vi "Page Engine.vi"(7 "Action":T5, 8 "error in (no error)":errorcluster, 11 "Data in":variant) -> (0 "error out":errorcluster, 3 "Data out":variant)   [LabVIEW 2018, in "Page.lvlib"]
uses:
  Page.lvlib
  Page Refnums.ctl
  Page Action.ctl
  Page Mouse.ctl
  <vilib>/Utility/miscctls.llb/LVPoint32TypeDef.ctl
  <vilib>/Utility/miscctls.llb/LVPointTypeDef.ctl
  Page Add.ctl
  Theme/Theme Colors.vi
  Theme/Theme.lvlib
  <vilib>/picture/picture.llb/imagedata.ctl
panel:
  in  "StateData":T4={"Refnums"={"VI Refnum"=refnum, "Sub Panel"=refnum, "Picture"=refnum}, "Page"={"Height"=32, "ActiveIdx"=0, "HoverIdx"=0, "Mouse"={"Horizontal"=0, "Vertical"=0, "Button"=0, "Shift"=FALSE, "Ctrl"=FALSE, "Alt"=FALSE, "Double Click"=FALSE}}, "Pages"={"VI Refnums"=[], "Captions"=[], "Titles"=[], "Images"=[], "Running"=[]}, "Ready"=FALSE}
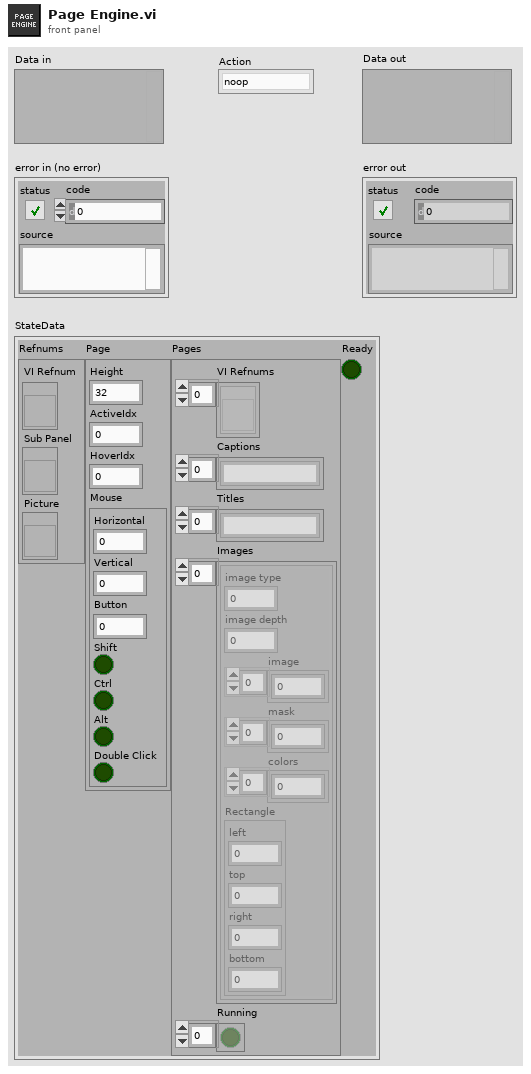
[diagram p1: front panel]
types:
  T1 = typedef "Page.lvlib/Page Refnums.ctl" = cluster{"VI Refnum":refnum<vi>, "Sub Panel":refnum<vi>, "Picture":refnum<vi>}
  T2 = typedef "Page.lvlib/Page Mouse.ctl" = cluster{"Horizontal":i32, "Vertical":i32, "Button":u16, "Shift":bool, "Ctrl":bool, "Alt":bool, "Double Click":bool}
  T3 = typedef "imagedata.ctl" = cluster{"image type":i32, "image depth":i32, "image":u8[], "mask":u8[], "colors":u32[], "Rectangle":cluster{"left":i16, "top":i16, "right":i16, "bottom":i16}}
  T4 = cluster{"Refnums":T1, "Page":cluster{"Height":i32, "ActiveIdx":i32, "HoverIdx":i32, "Mouse":T2}, "Pages":cluster{"VI Refnums":refnum<vi>[], "Captions":string[], "Titles":string[], "Images":T3[], "Running":bool[]}, "Ready":bool}
  T5 = typedef "Page.lvlib/Page Action.ctl" = enum8{"noop", "new", "init", "close", "page_change", "page_hover", "render", "page_caption", "page_insert", "page_add", "start", "resize", "theme_change", "hide"}
  T6 = typedef "LVPointTypeDef.ctl" = cluster{"Horizontal":i16, "Vertical":i16}
  T7 = typedef "LVPoint32TypeDef.ctl" = cluster{"Horizontal":i32, "Vertical":i32}
  T8 = cluster{"left":i16, "top":i16, "right":i16, "bottom":i16}
  T9 = typedef "Page.lvlib/Page Add.ctl" = cluster{"VI Path":path, "Caption":string}
  T10 = enum32{"Invalid", "Standard", "Closed", "Hidden", "Minimized", "Maximized"}
  T11 = typedef "LVRectTypeDef.ctl" = cluster{"Left":i16, "Top":i16, "Right":i16, "Bottom":i16}
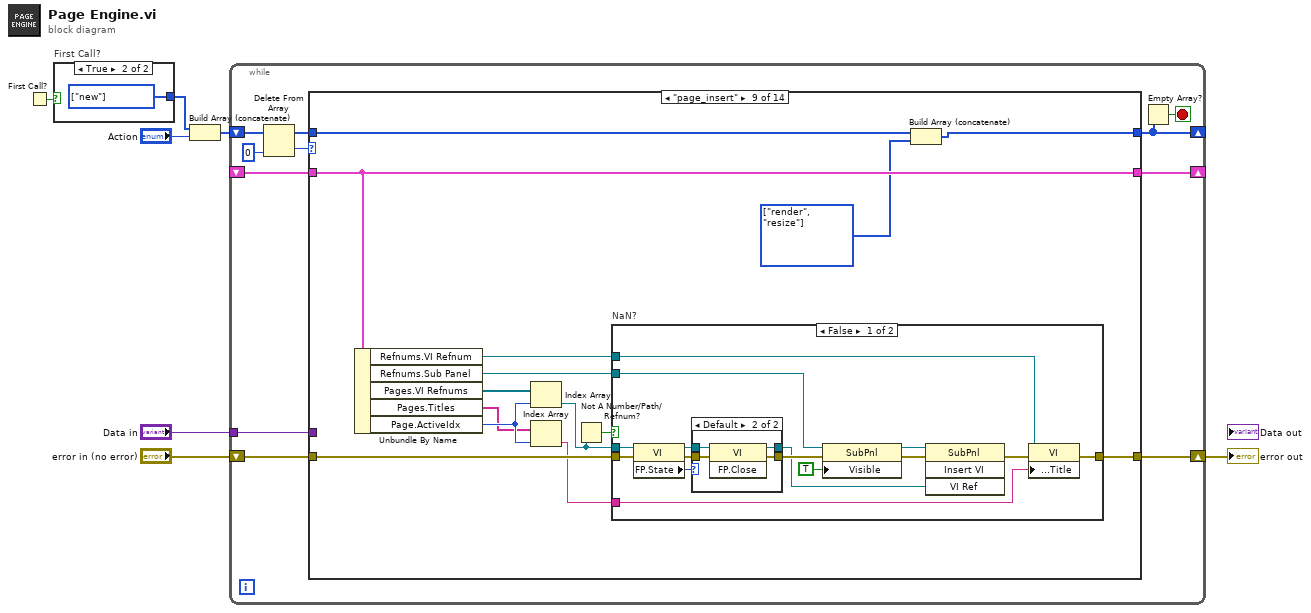
[diagram p0: block diagram]
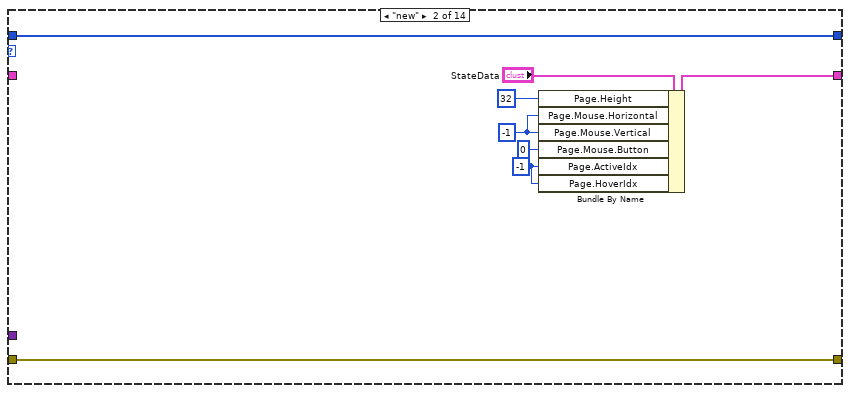
[diagram p4: hidden frame]
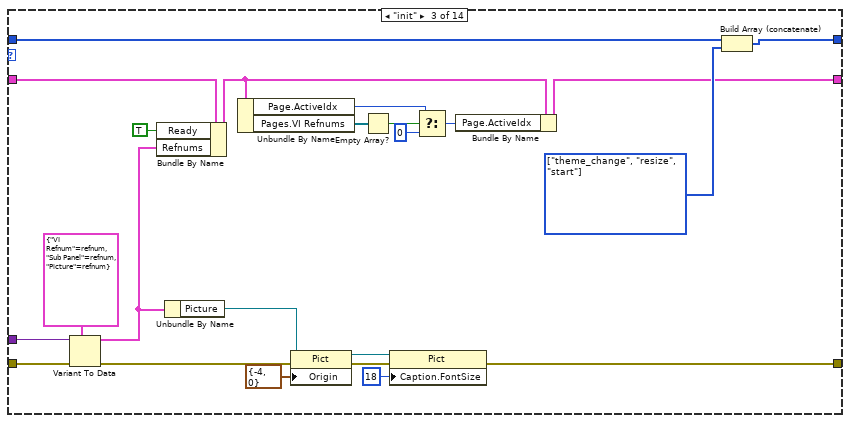
[diagram p5: hidden frame]
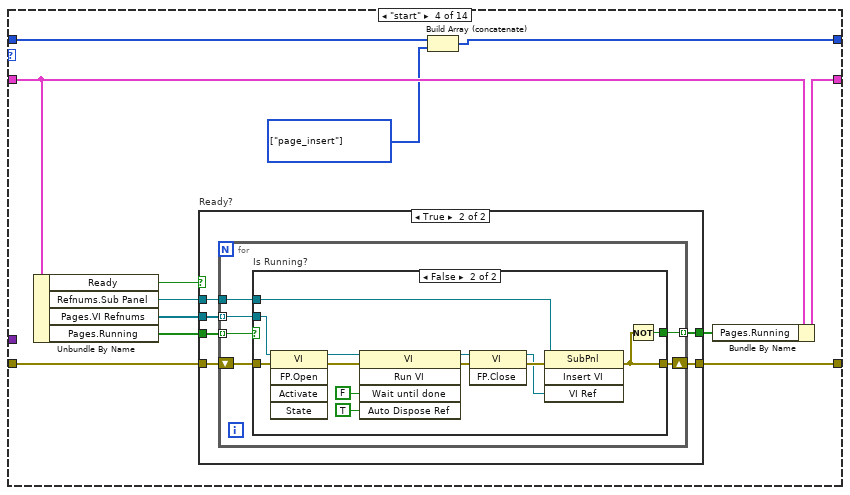
[diagram p6: hidden frame]
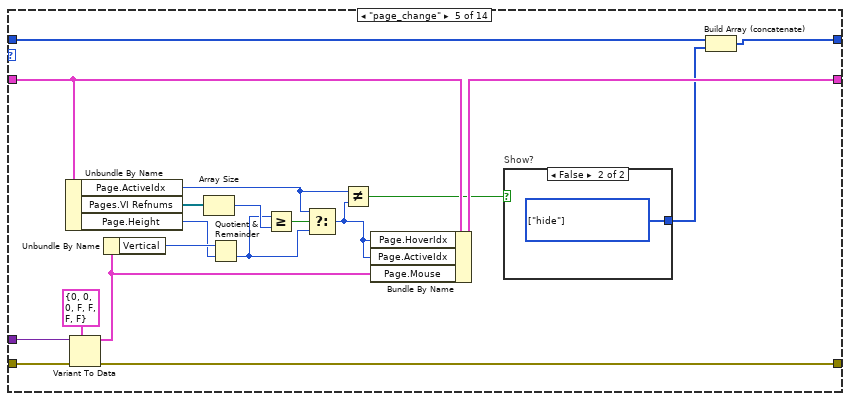
[diagram p9: hidden frame]
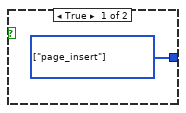
[diagram p10: hidden frame]
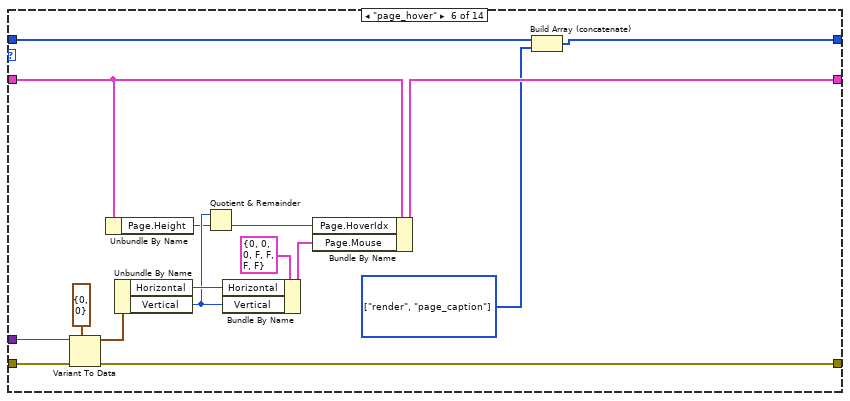
[diagram p11: hidden frame]
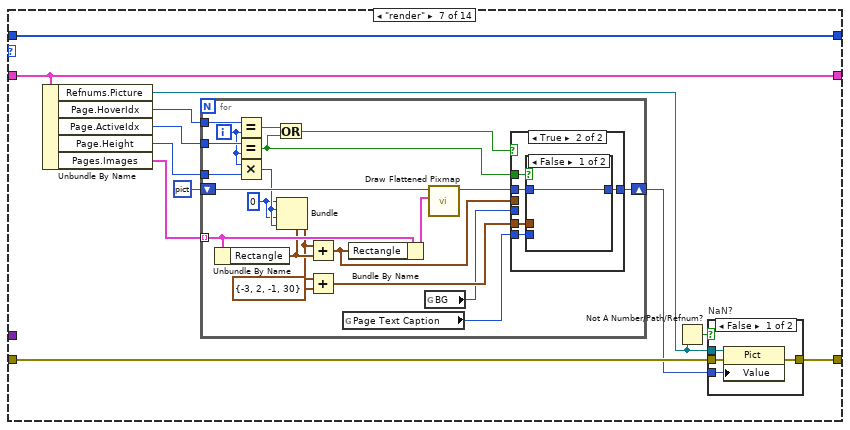
[diagram p12: hidden frame]
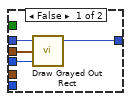
[diagram p14: hidden frame]
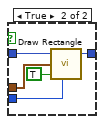
[diagram p15: hidden frame]
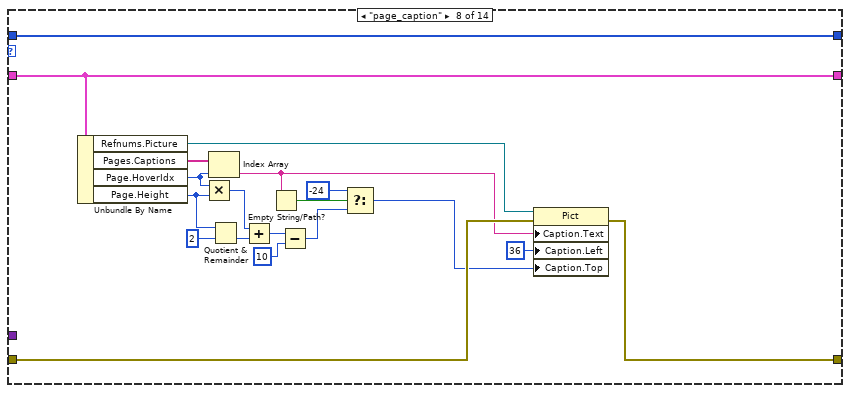
[diagram p16: hidden frame]
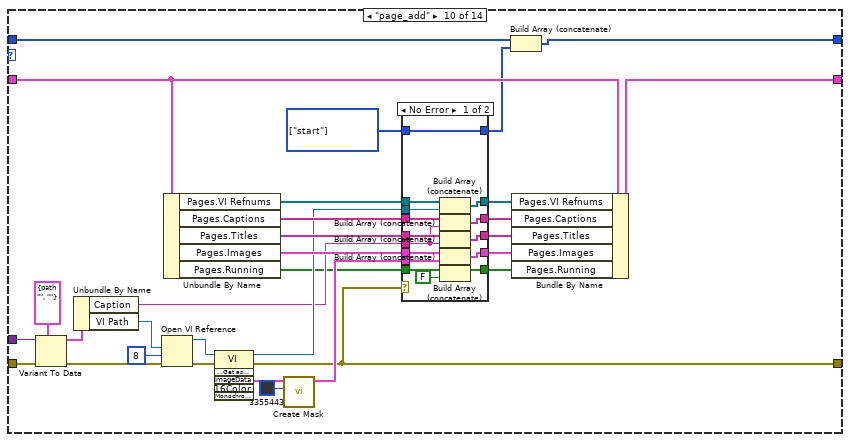
[diagram p19: hidden frame]
diagram:
  n1 = First Call?() -> (First Call?: T/F=w1:bool)
  n2 = case "First Call?" shown="True" w1 {
    tunnel: [_ w8] -> w2
    frame False {
    }
    frame True {
      w8 = T5[] [enum."new"] items=["noop", "new", "init", "close", "page_change", "page_hover", "render", "page_caption", "page_insert", "page_add", "start", "resize", "theme_change", "hide"] ("element")
    }
  }
  n3 = Build Array (concatenate)(w2, "Action") -> (w3:T5[])
  n4 = while {
    tunnel: "Data in" -> [w17]
    shift-right: [w18] -> w6
    shift-left: "error in (no error)" -> [w19]
    shift-right: [w12] -> _
    shift-left: w3 -> [w16]
    shift-right: [w10] -> _
    shift-left: _ -> [w9]
    stop <- w11 stop-if-true
    n5 = Delete From Array(array=w16, index=0) -> (deleted portion=w13:T5, array with subset deleted=w15:T5[])  [unwired: 1 in]
    n6 = case shown="\"page_insert\"" w13 {
      tunnel: w19 -> [w21 w30 w53 w62 w113 w131 w140 w196 w217 w270 w291 w317 w322 w362]
      tunnel: [w21 w30 w40 w63 w112 w130 w141 w197 w213 w248 w291 w306 w326 w355] -> w18
      tunnel: w17 -> [_ _ w51 _ w111 w129 _ _ _ w267 _ _ _ _]
      tunnel: w15 -> [w22 w29 w49 w65 w110 w128 w143 w203 w216 w269 w293 w316 w328 w361]
      tunnel: [w22 w29 w47 w58 w108 w126 w143 w203 w211 w247 w293 w316 w319 w358] -> w12
      tunnel: [w20 w27 w32 w55 w109 w127 w142 w202 w215 w262 w292 w315 w327 w360] -> w10
      tunnel: w9 -> [w20 _ w48 w64 w104 w124 w142 w202 w215 w263 w292 w315 w327 w356]
      frame "noop" {
      }
      frame "new" {
        w23 = -1 ("Page.ActiveIdx")
        w25 = -1 ("Page Mouse.Vertical")
        n7 = Bundle By Name(cluster="StateData", "Page.Height"=32 ("PageHeight"), "Page.Mouse.Horizontal"=w25, "Page.Mouse.Vertical"=w25, "Page.Mouse.Button"=u16 0, "Page.ActiveIdx"=w23, "Page.HoverIdx"=w23) -> (w27:T4)
      }
      frame "init" {
        w46 = T5[] [enum."theme_change", enum."resize", enum."start"] items=["noop", "new", "init", "close", "page_change", "page_hover", "render", "page_caption", "page_insert", "page_add", "start", "resize", "theme_change", "hide"] ("array")
        n8 = Variant To Data(error in=w53, type=T1 {"VI Refnum"=refnum, "Sub Panel"=refnum, "Picture"=refnum} ("Refnums"), Variant=w51) -> (data=w45:T1, error out=w52:errorcluster)
        n9 = Bundle By Name(cluster=w48, "Ready"=TRUE, "Refnums"=w45) -> (w37:T4)
        n10 = Unbundle By Name(w45) -> ("Picture"=w43:refnum<vi>)
        n11 = Unbundle By Name(w37) -> ("Page.ActiveIdx"=w34:i32, "Pages.VI Refnums"=w36:refnum<vi>[])
        n12 = property class="Pict"(reference=w43, error in=w52, "Origin"=T6 {"Horizontal"=-4, "Vertical"=0}) -> (reference out=w39:refnum<vi>, error out=w44:errorcluster)
        n13 = Empty Array?(array=w36) -> (empty?=w35:bool)
        n14 = property class="Pict"(reference=w39, error in=w44, "Caption.FontSize"=u32 18 ("Caption.Font:Size")) -> (error out=w40:errorcluster)  [unwired: 1 out]
        n15 = Select(t=w34, s=w35, f=0) -> (s? t:f=w31:i32)
        n16 = Bundle By Name(cluster=w37, "Page.ActiveIdx"=w31) -> (w32:T4)
        n17 = Build Array (concatenate)(w49, w46) -> (w47:T5[])
      }
      frame "start" {
        w57 = T5[] [enum."page_insert"] items=["noop", "new", "init", "close", "page_change", "page_hover", "render", "page_caption", "page_insert", "page_add", "start", "resize", "theme_change", "hide"] ("array")
        n18 = Unbundle By Name(w64) -> ("Ready"=w59:bool, "Refnums.Sub Panel"=w60:refnum<vi>, "Pages.VI Refnums"=w61:refnum<vi>[], "Pages.Running"=w56:bool[])
        n19 = case "Ready?" shown="True" w59 {
          tunnel: [w67 w73] -> w63
          tunnel: w62 -> [w67 w72]
          tunnel: w61 -> [_ w71]
          tunnel: w60 -> [_ w70]
          tunnel: w56 -> [w66 w69]
          tunnel: [w66 w68] -> w54
          frame False {
          }
          frame True {
            n20 = for {
              tunnel: w71 -> [w77] mode=indexing
              shift-right: [w79] -> w73
              shift-left: w72 -> [w76]
              tunnel: w70 -> [w78]
              tunnel: w69 -> [w75] mode=indexing
              tunnel: [w74] -> w68 mode=indexing
              n21 = case "Is Running?" shown="False" w75 {
                selector: w75 -> [w80 _]
                tunnel: w76 -> [w81 w87]
                tunnel: w77 -> [_ w86]
                tunnel: [w81 w83] -> w79
                tunnel: w78 -> [_ w85]
                tunnel: [w80 w82] -> w74
                frame True {
                }
                frame False {
                  n22 = invoke class="VI" method="FP.Open"(reference=w86, error in=w87) -> (reference out=w90:refnum<vi>, error out=w91:errorcluster)  [unwired: 3 in, 3 out]
                  n23 = invoke class="VI" method="Run VI"(reference=w90, error in=w91, "Wait until done"=FALSE ("Wait Until Done"), "Auto Dispose Ref"=TRUE ("Auto Dispose Reference")) -> (reference out=w89:refnum<vi>, error out=w94:errorcluster)  [unwired: 1 in, 3 out]
                  n24 = invoke class="VI" method="FP.Close"(reference=w89, error in=w94) -> (reference out=w84:refnum<vi>, error out=w88:errorcluster)  [unwired: 1 in, 1 out]
                  n25 = invoke class="SubPnl" method="Insert VI"(reference=w85, error in=w88, "VI Ref"=w84) -> (error out=w83:errorcluster)  [unwired: 1 in, 3 out]
                  n26 = Not(x=w83) -> (.not. x?=w82:bool)
                }
              }
            }
          }
        }
        n27 = Build Array (concatenate)(w65, w57) -> (w58:T5[])
        n28 = Bundle By Name(cluster=w64, "Pages.Running"=w54) -> (w55:T4)
      }
      frame "page_change" {
        n29 = Unbundle By Name(w104) -> ("Page.ActiveIdx"=w96:i32, "Pages.VI Refnums"=w101:refnum<vi>[], "Page.Height"=w102:i32)
        n30 = Variant To Data(error in=w113, type=T2 {"Horizontal"=0, "Vertical"=0, "Button"=0, "Shift"=FALSE, "Ctrl"=FALSE, "Alt"=FALSE, "Double Click"=FALSE} ("Page Mouse"), Variant=w111) -> (data=w105:T2, error out=w112:errorcluster)
        n31 = Unbundle By Name(w105) -> ("Vertical"=w103:i32)
        n32 = Array Size(array=w101) -> (size(s)=w100:i32)
        n33 = Quotient & Remainder(x=w103, y=w102) -> (floor(x/y)=w98:i32)  [unwired: 1 out]
        n34 = Greater Or Equal?(x=w98, y=w100) -> (x >= y?=w99:bool)
        n35 = Select(t=w96, s=w99, f=w98) -> (s? t:f=w97:i32)
        n36 = Not Equal?(x=w96, y=w97) -> (x != y?=w95:bool)
        n37 = Bundle By Name(cluster=w104, "Page.HoverIdx"=w97, "Page.ActiveIdx"=w97, "Page.Mouse"=w105) -> (w109:T4)
        n38 = case "Show?" shown="False" w95 {
          tunnel: [w114 w115] -> w107
          frame True {
            w114 = T5[] [enum."page_insert"] items=["noop", "new", "init", "close", "page_change", "page_hover", "render", "page_caption", "page_insert", "page_add", "start", "resize", "theme_change", "hide"] ("array")
          }
          frame False {
            w115 = T5[] [enum."hide"] items=["noop", "new", "init", "close", "page_change", "page_hover", "render", "page_caption", "page_insert", "page_add", "start", "resize", "theme_change", "hide"] ("array")
          }
        }
        n39 = Build Array (concatenate)(w110, w107) -> (w108:T5[])
      }
      frame "page_hover" {
        w125 = T5[] [enum."render", enum."page_caption"] items=["noop", "new", "init", "close", "page_change", "page_hover", "render", "page_caption", "page_insert", "page_add", "start", "resize", "theme_change", "hide"] ("array")
        n40 = Variant To Data(error in=w131, type=T7 {"Horizontal"=0, "Vertical"=0} ("Coords"), Variant=w129) -> (data=w120:T7, error out=w130:errorcluster)
        n41 = Unbundle By Name(w124) -> ("Page.Height"=w117:i32)
        n42 = Unbundle By Name(w120) -> ("Horizontal"=w119:i32, "Vertical"=w118:i32)
        n43 = Quotient & Remainder(x=w118, y=w117) -> (floor(x/y)=w116:i32)  [unwired: 1 out]
        n44 = Bundle By Name(cluster=T2 {"Horizontal"=0, "Vertical"=0, "Button"=0, "Shift"=FALSE, "Ctrl"=FALSE, "Alt"=FALSE, "Double Click"=FALSE} ("Page.Mouse"), "Horizontal"=w119, "Vertical"=w118) -> (w122:T2)
        n45 = Bundle By Name(cluster=w124, "Page.HoverIdx"=w116, "Page.Mouse"=w122) -> (w127:T4)
        n46 = Build Array (concatenate)(w128, w125) -> (w126:T5[])
      }
      frame "render" {
        n47 = Unbundle By Name(w142) -> ("Refnums.Picture"=w133:refnum<vi>, "Page.HoverIdx"=w137:i32, "Page.ActiveIdx"=w138:i32, "Page.Height"=w135:i32, "Pages.Images"=w139:T3[])
        n48 = for {
          tunnel: w139 -> [w168] mode=indexing
          tunnel: w138 -> [w169]
          tunnel: w137 -> [w166]
          shift-right: [w164] -> w134
          shift-left: picture data[5B] ("new picture") -> [w163]
          tunnel: w135 -> [w160]
          i -> [w161]
          w157 = i16 0 ("left")
          n49 = Unbundle By Name(w168) -> ("Rectangle"=w162:T8)
          n50 = Equal?(x=w166, y=w161) -> (x = y?=w158:bool)
          n51 = Equal?(x=w169, y=w161) -> (x = y?=w151:bool)
          n52 = Multiply(x=w161, y=w160) -> (x*y=w159:i32)
          n53 = Or(x=w158, y=w151) -> (x .or. y?=w152:bool)
          n54 = Bundle(cluster=w162, "left"=w157, "top"=w159, "right"=w157, "bottom"=w159) -> (w155:T8)
          n55 = Add(x=w155, y=w162) -> (x+y=w156:T8)
          n56 = Add(x=w155, y=T8 {"left"=-3, "top"=2, "right"=-1, "bottom"=30}) -> (x+y=w153:T8)
          n57 = global read "Theme Colors.vi" "Page Text Caption"() -> (w149:u32)
          n58 = Bundle By Name(cluster=w168, "Rectangle"=w156) -> (w167:T3)
          n59 = global read "Theme Colors.vi" "BG"() -> (w150:u32)
          n60 = call <vilib>:"Draw Flattened Pixmap.vi"("image data"=w167, "picture"=w163) -> ("new picture"=w165:picture)  [unwired: 7 in]
          n61 = case shown="True" w152 {
            tunnel: w150 -> [w173 _]
            tunnel: w165 -> [w172 w178]
            tunnel: w156 -> [w171 _]
            tunnel: [w170 w177] -> w164
            tunnel: w153 -> [_ w176]
            tunnel: w149 -> [_ w175]
            tunnel: w151 -> [_ w174]
            frame False {
              n62 = call <vilib>:"Draw Grayed Out Rect.vi"("color(black)"=w173, "rect"=w171, "picture"=w172) -> ("new picture"=w170:picture)  [unwired: 2 in]
            }
            frame True {
              n63 = case shown="False" w174 {
                tunnel: w178 -> [w179 w184]
                tunnel: [w179 w183] -> w177
                tunnel: w176 -> [_ w182]
                tunnel: w175 -> [_ w180]
                frame False {
                }
                frame True {
                  n64 = call <vilib>:"Draw Rectangle.vi"("picture"=w184, "rect"=w182, "fill?(F)"=TRUE, "color(black)"=w180) -> ("new picture"=w183:picture)  [unwired: 5 in]
                }
              }
            }
          }
        }
        n65 = Not A Number/Path/Refnum?(number/path/refnum=w133) -> (NaN/Path/Refnum?=w132:bool)
        n66 = case "NaN?" shown="False" w132 {
          tunnel: w133 -> [w147 _]
          tunnel: [w146 w148] -> w141
          tunnel: w140 -> [w145 w148]
          tunnel: w134 -> [w144 _]
          frame False {
            n67 = property class="Pict"(reference=w147, error in=w145, "Value"=w144) -> (error out=w146:errorcluster)  [unwired: 1 out]
          }
          frame True {
          }
        }
      }
      frame "page_caption" {
        n68 = Unbundle By Name(w202) -> ("Refnums.Picture"=w201:refnum<vi>, "Pages.Captions"=w200:string[], "Page.HoverIdx"=w198:i32, "Page.Height"=w192:i32)
        n69 = Multiply(x=w198, y=w192) -> (x*y=w189:i32)
        n70 = Index Array(array=w200, index=w198) -> (element=w195:string)
        n71 = Quotient & Remainder(x=w192, y=2) -> (floor(x/y)=w187:i32)  [unwired: 1 out]
        n72 = Add(x=w189, y=w187) -> (x+y=w186:i32)
        n73 = Empty String/Path?(string/path=w195) -> (empty?=w194:bool)
        n74 = Subtract(x=w186, y=10) -> (x-y=w185:i32)
        n75 = Select(t=-24, s=w194, f=w185) -> (s? t:f=w190:i32)
        n76 = property class="Pict"(reference=w201, error in=w196, "Caption.Text"=w195, "Caption.Left"=36 ("Caption.Position:Left"), "Caption.Top"=w190) -> (error out=w197:errorcluster)  [unwired: 1 out]
      }
      frame "page_insert" {
        w210 = T5[] [enum."render", enum."resize"] items=["noop", "new", "init", "close", "page_change", "page_hover", "render", "page_caption", "page_insert", "page_add", "start", "resize", "theme_change", "hide"] ("array")
        n77 = Unbundle By Name(w215) -> ("Refnums.VI Refnum"=w205:refnum<vi>, "Refnums.Sub Panel"=w214:refnum<vi>, "Pages.VI Refnums"=w212:refnum<vi>[], "Pages.Titles"=w206:string[], "Page.ActiveIdx"=w207:i32)
        n78 = Index Array(array=w212, index=w207) -> (element=w209:refnum<vi>)
        n79 = Index Array(array=w206, index=w207) -> (element=w204:string)
        n80 = Not A Number/Path/Refnum?(number/path/refnum=w209) -> (NaN/Path/Refnum?=w208:bool)
        n81 = case "NaN?" shown="False" w208 {
          tunnel: w217 -> [w232 w239]
          tunnel: w214 -> [w219 _]
          tunnel: [w224 w239] -> w213
          tunnel: w209 -> [w226 _]
          tunnel: w205 -> [w223 _]
          tunnel: w204 -> [w222 _]
          frame False {
            n82 = property class="VI"(reference=w226, error in=w232) -> (reference out=w228:refnum<vi>, error out=w230:errorcluster, "FP.State"=w227:T10)
            n83 = case shown="Default" w227 {
              tunnel: w230 -> [w234 w238]
              tunnel: [w234 w237] -> w229
              tunnel: w228 -> [w233 w236]
              tunnel: [w233 w235] -> w225
              frame "Invalid", "Closed" {
              }
              frame Default {
                n84 = invoke class="VI" method="FP.Close"(reference=w236, error in=w238) -> (reference out=w235:refnum<vi>, error out=w237:errorcluster)  [unwired: 1 in, 1 out]
              }
            }
            n85 = property class="SubPnl"(reference=w219, error in=w229, "Visible"=TRUE) -> (reference out=w220:refnum<vi>, error out=w221:errorcluster)
            n86 = invoke class="SubPnl" method="Insert VI"(reference=w220, error in=w221, "VI Ref"=w225) -> (error out=w231:errorcluster)  [unwired: 1 in, 3 out]
            n87 = property class="VI"(reference=w223, error in=w231, "Front Panel.Title"=w222) -> (error out=w224:errorcluster)  [unwired: 1 out]
          }
          frame True {
          }
        }
        n88 = Build Array (concatenate)(w216, w210) -> (w211:T5[])
      }
      frame "page_add" {
        w245 = T5[] [enum."start"] items=["noop", "new", "init", "close", "page_change", "page_hover", "render", "page_caption", "page_insert", "page_add", "start", "resize", "theme_change", "hide"] ("array")
        n89 = Variant To Data(error in=w270, type=T9 {"VI Path"=path "", "Caption"=""} ("Page Add"), Variant=w267) -> (data=w266:T9, error out=w268:errorcluster)
        n90 = Unbundle By Name(w266) -> ("Caption"=w249:string, "VI Path"=w265:path)
        n91 = Open VI Reference(vi path=w265, options=8, error in (no error)=w268) -> (vi reference=w242:refnum<vi>, error out=w243:errorcluster)  [unwired: 3 in]
        n92 = Unbundle By Name(w263) -> ("Pages.VI Refnums"=w261:refnum<vi>[], "Pages.Captions"=w260:string[], "Pages.Titles"=w259:string[], "Pages.Images"=w258:T3[], "Pages.Running"=w241:bool[])
        n93 = invoke class="VI" method="VI Icon.Get as Image Data"(reference=w242, error in=w243) -> (reference out=w250:refnum<vi>, error out=w248:errorcluster, "ImageData"=w253:T3)  [unwired: 4 in, 3 out]
        n94 = call <vilib>:"Create Mask.vi"("Mask Color (Black)"=u32 3355443, "image data"=w253) -> ("image data"=w251:T3)  [unwired: 9 in]
        n95 = case shown="No Error" w248 {
          tunnel: w261 -> [w274 w290]
          tunnel: w260 -> [w285 w289]
          tunnel: w259 -> [w284 w288]
          tunnel: w258 -> [w283 w287]
          tunnel: [w282 w287] -> w257
          tunnel: [w281 w288] -> w256
          tunnel: [w280 w289] -> w255
          tunnel: [w279 w290] -> w254
          tunnel: w251 -> [w278 _]
          tunnel: w250 -> [w277 _]
          tunnel: w249 -> [w276 _]
          tunnel: [w275 _] -> w246
          tunnel: w245 -> [w275 _]
          tunnel: w241 -> [w273 w286]
          tunnel: [w272 w286] -> w240
          frame No Error {
            n96 = Build Array (concatenate)(w274, w277) -> (w279:refnum<vi>[])
            n97 = Build Array (concatenate)(w285, w276) -> (w280:string[])
            n98 = Build Array (concatenate)(w284, w276) -> (w281:string[])
            n99 = Build Array (concatenate)(w283, w278) -> (w282:T3[])
            n100 = Build Array (concatenate)(w273, FALSE ("element")) -> (w272:bool[])
          }
          frame Error {
          }
        }
        n101 = Build Array (concatenate)(w269, w246) -> (w247:T5[])
        n102 = Bundle By Name(cluster=w263, "Pages.VI Refnums"=w254, "Pages.Captions"=w255, "Pages.Titles"=w256, "Pages.Images"=w257, "Pages.Running"=w240) -> (w262:T4)
      }
      frame "close" {
      }
      frame "resize" {
        w298 = 36 ("Position:Left")
        n103 = Unbundle By Name(w315) -> ("Refnums.Sub Panel"=w295:refnum<vi>, "Refnums.VI Refnum"=w313:refnum<vi>)
        n104 = property class="VI"(reference=w313, error in=w317) -> (error out=w314:errorcluster, "Panel"=w311:refnum<vi>)  [unwired: 1 out]
        n105 = property class="Pnl"(reference=w311, error in=w314) -> (error out=w312:errorcluster, "Panes[]"=w310:refnum<vi>[])  [unwired: 1 out]
        n106 = Index Array(array=w310) -> (element=w308:refnum<vi>)  [unwired: 1 in]
        n107 = property class="Pane"(reference=w308, error in=w312) -> (error out=w309:errorcluster, "ContentBnds"=w307:T11)  [unwired: 1 out]
        n108 = Unbundle By Name(w307) -> ("Right"=w302:i16, "Left"=w301:i16, "Bottom"=w304:i16, "Top"=w303:i16)
        n109 = Subtract(x=w302, y=w301) -> (x-y=w300:i16)
        n110 = Subtract(x=w304, y=w303) -> (x-y=w296:i16)
        n111 = Subtract(x=w300, y=w298) -> (x-y=w299:i32)
        n112 = Subtract(x=w299, y=3) -> ()  [unwired: 1 out]
        n113 = property class="SubPnl"(reference=w295, error in=w309, "Left"=w298, "Top"=-3 ("Position:Top"), "Width"=u32 252 ("Container Bounds:Width"), "Height"=w296) -> (error out=w306:errorcluster)  [unwired: 1 out]
      }
      frame "theme_change" {
        w318 = T5[] [enum."render"] items=["noop", "new", "init", "close", "page_change", "page_hover", "render", "page_caption", "page_insert", "page_add", "start", "resize", "theme_change", "hide"] ("array")
        n114 = Unbundle By Name(w327) -> ("Refnums.Picture"=w325:refnum<vi>, "Refnums.VI Refnum"=w320:refnum<vi>)
        n115 = Not A Number/Path/Refnum?(number/path/refnum=w320) -> (NaN/Path/Refnum?=w323:bool)
        n116 = case "NaN?" shown="False" w323 {
          tunnel: [w330 w346] -> w321
          tunnel: w322 -> [w339 w346]
          tunnel: w320 -> [w338 _]
          frame False {
            n117 = property class="VI"(reference=w338, error in=w339) -> (error out=w340:errorcluster, "Panel"=w336:refnum<vi>)  [unwired: 1 out]
            n118 = property class="Pnl"(reference=w336, error in=w340) -> (reference out=w329:refnum<vi>, error out=w337:errorcluster, "Panes[]"=w334:refnum<vi>[])
            n119 = global read "Theme Colors.vi" "BG"() -> (w333:u32)
            n120 = for {
              tunnel: w334 -> [w343] mode=indexing
              shift-right: [w344] -> w335
              shift-left: w337 -> [w345]
              tunnel: w333 -> [w342]
              tunnel: [w341] -> w331 mode=indexing
              n121 = property class="Pane"(reference=w343, error in=w345, "PaneColor"=w342) -> (reference out=w341:refnum<vi>, error out=w344:errorcluster)
            }
            n122 = Close Reference(reference=w331, error in (no error)=w335) -> (error out=w332:errorcluster)
            n123 = Close Reference(reference=w329, error in (no error)=w332) -> (error out=w330:errorcluster)
          }
          frame True {
          }
        }
        n124 = Build Array (concatenate)(w328, w318) -> (w319:T5[])
        n125 = Not A Number/Path/Refnum?(number/path/refnum=w325) -> (NaN/Path/Refnum?=w324:bool)
        n126 = case "NaN?" shown="False" w324 {
          tunnel: [w349 w352] -> w326
          tunnel: w321 -> [w348 w352]
          tunnel: w325 -> [w347 _]
          frame False {
            n127 = global read "Theme Colors.vi" "Page Text Caption"() -> (w351:u32)
            n128 = global read "Theme Colors.vi" "BG"() -> (w350:u32)
            n129 = property class="Pict"(reference=w347, error in=w348, "Caption.TextColor"=w351, "Caption.BG Color"=w350) -> (error out=w349:errorcluster)  [unwired: 1 out]
          }
          frame True {
          }
        }
      }
      frame "hide" {
        w357 = T5[] [enum."render"] items=["noop", "new", "init", "close", "page_change", "page_hover", "render", "page_caption", "page_insert", "page_add", "start", "resize", "theme_change", "hide"] ("array")
        n130 = Unbundle By Name(w356) -> ("Refnums.Sub Panel"=w354:refnum<vi>)
        n131 = property class="SubPnl"(reference=w354, error in=w362, "Visible"=FALSE) -> (error out=w355:errorcluster)  [unwired: 1 out]
        n132 = Bundle By Name(cluster=w356, "Page.ActiveIdx"=-1) -> (w360:T4)
        n133 = Build Array (concatenate)(w361, w357) -> (w358:T5[])
      }
    }
    n134 = Empty Array?(array=w12) -> (empty?=w11:bool)
  }
  "error out" <- w6
